vi "Adjust for Camera offset.vi"(2 "Distance":dbl, 3 "Angle":dbl) -> (0 "Distance":dbl, 1 "Angle":dbl)   [LabVIEW 2018]
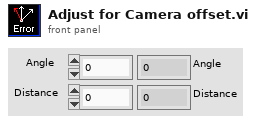
[diagram p1: front panel]
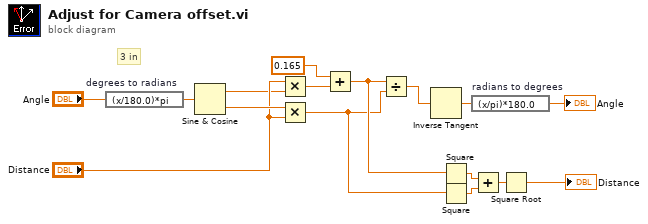
[diagram p0: block diagram]
diagram:
  # "3 in"
  n1 = expression code="(x/180.0)*pi" "degrees to radians"("Angle") -> (w15:dbl)
  n2 = Sine & Cosine(0:w15) -> (1:w1:dbl, 2:w14:dbl)
  n3 = Multiply(x="Distance", y=w1) -> (x*y=w12:dbl)
  n4 = Multiply(x=w14, y="Distance") -> (x*y=w6:dbl)
  n5 = Add(x=0.165, y=w12) -> (x+y=w7:dbl)
  n6 = Divide(x=w7, y=w6) -> (x/y=w9:dbl)
  n7 = Inverse Tangent(1:w9) -> (0:w8:dbl)
  n8 = Square(x=w7) -> (x^2=w4:dbl)
  n9 = Square(x=w6) -> (x^2=w5:dbl)
  n10 = expression code="(x/pi)*180.0" "radians to degrees"(w8) -> (→"Angle":dbl)
  n11 = Add(x=w4, y=w5) -> (x+y=w3:dbl)
  n12 = Square Root(x=w3) -> (sqrt(x)=→"Distance":dbl)
